vi "MAG ON.vi"(8 "error in (no error)":errorcluster, 9 "PSU Status In":T1 {"Trip Current" format="%.3f"; "Trip Field" format="%.4f"; "Voltage" format="%.2f"; "Field Constant" format="%.6f"; "MID Setpoint (T)" format="%.4f"; "MID Setpoint (A)" format="%.3f"; "MAX Setpoint (T)" format="%.4f"; "MAX Setpoint (A)" format="%.3f"; "Heater Voltage" format="%.2f"; "V Limit (V)" format="%.2f"; "Ramp Rate (A/s)" format="%.3f"; "Output (A)" format="%.3f"; "Output (T)" format="%.4f"; "Persistent Current" format="%.3f"; "Persistent Field" format="%.4f"}, 10 "MagQ in":refnum<queue>, 11 "VISA Refnum in":refnum<visa-resource-name>) -> (0 "error out":errorcluster, 1 "PSU Status Out":T1 {"Trip Current" format="%.3f"; "Trip Field" format="%.4f"; "Voltage" format="%.2f"; "Field Constant" format="%.6f"; "MID Setpoint (T)" format="%.4f"; "MID Setpoint (A)" format="%.3f"; "MAX Setpoint (T)" format="%.4f"; "MAX Setpoint (A)" format="%.3f"; "Heater Voltage" format="%.2f"; "V Limit (V)" format="%.2f"; "Ramp Rate (A/s)" format="%.3f"; "Output (A)" format="%.3f"; "Output (T)" format="%.4f"; "Persistent Current" format="%.3f"; "Persistent Field" format="%.4f"}, 2 "MagQ out":refnum<queue>, 3 "VISA Refnum out":refnum<visa-resource-name>, 5 "MID Setpoint (T)":dbl)   [LabVIEW 2025]
uses:
  <instrlib>/SMS LabVIEW Drivers/Source Code/Public/PSU Status.ctl
  <instrlib>/SMS LabVIEW Drivers/Source Code/Cryogenic Ltd SMSXXX.lvlib
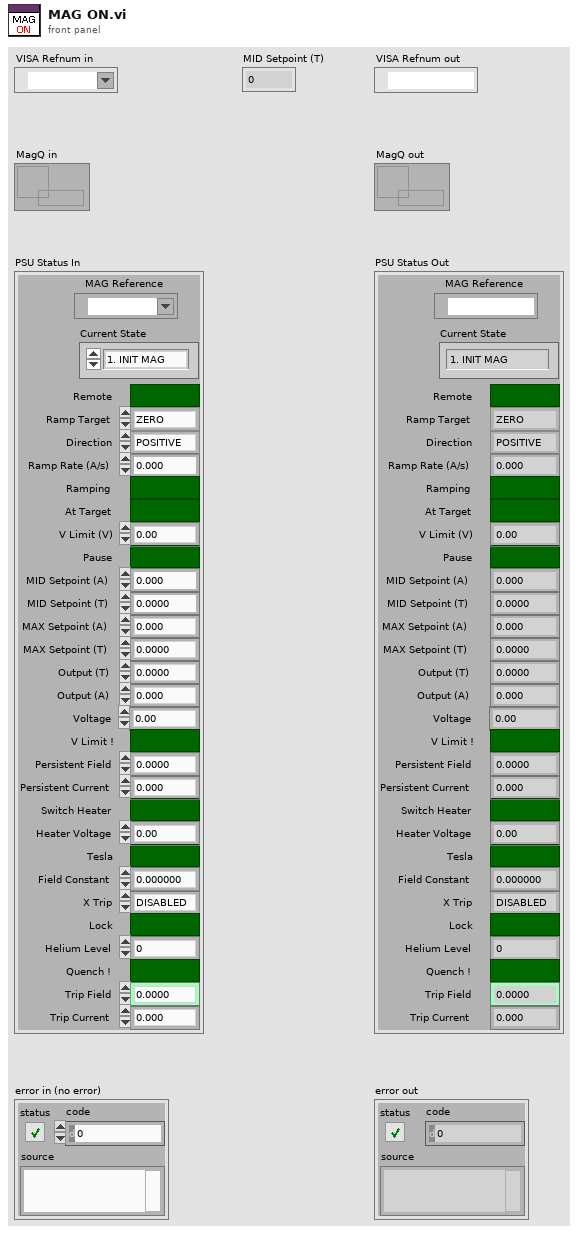
[diagram p1: front panel]
types:
  T1 = typedef "PSU Status.ctl" = cluster{"Ramp Target":enum16{"ZERO", "MID", "MAX"}, "Pause":bool, "Switch Heater":bool, "Persistent Field":dbl, "Persistent Current":dbl, "Tesla":bool, "Output (T)":dbl, "Output (A)":dbl, "X Trip":enum16{"DISABLED", "ENABLED", "ACTIVE"}, "Ramp Rate (A/s)":dbl, "V Limit (V)":dbl, "Heater Voltage":dbl, "MAX Setpoint (A)":dbl, "MAX Setpoint (T)":dbl, "MID Setpoint (A)":dbl, "MID Setpoint (T)":dbl, "Lock":bool, "Field Constant":dbl, "Remote":bool, "Direction":enum16{"POSITIVE", "NEGATIVE", "OPEN", "UNIPOLAR"}, "Helium Level":u16, "Quench !":bool, "Voltage":dbl, "V Limit !":bool, "Ramping":bool, "At Target":bool, "Trip Field":dbl, "Trip Current":dbl, "Current State":enum16{"1. INIT MAG", "2. MAG ON", "3. MAG_STAB", "4. MAG IDLE", "5. PREP NEXT FIELD", "6. APPLY NEXT FIELD", "7. PREP OFF", "8. MAG OFF (Reset)"}, "MAG Reference":refnum<visa-resource-name>}
  T2 = enum16{"1. INIT MAG", "2. MAG ON", "3. MAG_STAB", "4. MAG IDLE", "5. PREP NEXT FIELD", "6. APPLY NEXT FIELD", "7. PREP OFF", "8. MAG OFF (Reset)"}
  T3 = enum16{"RAMP TO ZERO", "RAMP TO MID", "RAMP TO MAX"}
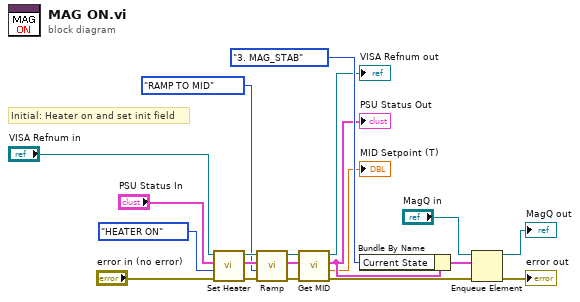
[diagram p0: block diagram]
diagram:
  # "Initial: Heater on and set init field"
  n1 = call <instrlib>:"Set Heater.vi"("Error in (no error)"="error in (no error)", "Heater (On/Off)"=enum16{"HEATER OFF", "HEATER ON"}."HEATER ON", "PSU Status In"="PSU Status In", "VISA Resource Name In"="VISA Refnum in") -> ("Error out"=w10:errorcluster, "PSU Status Out"=w11:T1, "VISA Resource Name Out"=w9:refnum<visa-resource-name>)  [unwired: 4 in, 1 out]
  n2 = call <instrlib>:"Ramp.vi"("Error in (no error)"=w10, "Ramp Target"=T3."RAMP TO MID", "PSU Status In"=w11, "VISA Resource Name In"=w9) -> ("Error out"=w4:errorcluster, "PSU Status Out"=w3:T1, "VISA Resource Name Out"=w2:refnum<visa-resource-name>)  [unwired: 4 in, 1 out]
  n3 = call <instrlib>:"Get MID.vi"("Error in (no error)"=w4, "PSU Status In"=w3, "VISA Resource Name In"=w2) -> ("Error out"=w16:errorcluster, "MID Setpoint (T)"=→"MID Setpoint (T)":dbl, "PSU Status Out"=w15:T1, "VISA Resource Name Out"=→"VISA Refnum out":refnum<visa-resource-name>)  [unwired: 3 in, 2 out]
  "PSU Status Out" <- w15
  n4 = Bundle By Name(cluster=w15, "Current State"=T2."3. MAG_STAB") -> (w14:T1)
  n5 = Enqueue Element(queue="MagQ in", element=w14, error in (no error)=w16) -> (queue out=→"MagQ out":refnum<queue>, error out=→"error out":errorcluster)  [unwired: 1 in, 1 out]
